vi "Format Log Message on Single Line.vi"(11 "Log Message":string) -> (3 "Formatted Log Message":string)   [LabVIEW 2020, in "WSsupport.lvlib"]
uses:
  WSsupport.lvlib
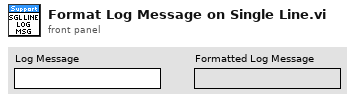
[diagram p1: front panel]
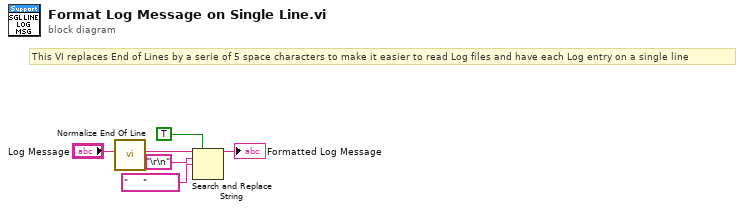
[diagram p0: block diagram]
diagram:
  # "This VI replaces End of Lines by a serie of 5 space characters to make it easier to read Log files and have each Log entry on a single line"
  n1 = call <vilib>:"Normalize End Of Line.vi"("string in"="Log Message") -> ("string out"=w4:string)  [unwired: 7 in]
  n2 = Search and Replace String(replace all?=TRUE ("replace all? (F)"), input string=w4, search string="\r\n", replace string="     " ("replace string (\"\")")) -> (result string=→"Formatted Log Message":string)  [unwired: 4 in, 3 out]
